vi "GetTau Delay ms.vi"(8 "error in (no error)":errorcluster, 11 "reference in":refnum<class "Force Curve_tdms.lvclass">) -> (0 "error out":errorcluster, 2 "Tau Delay ms":dbl=2.0 format="%#_13g", 3 "reference out":refnum<class "Force Curve_tdms.lvclass">)   [LabVIEW 2019, in "Force Curve_tdms.lvclass"]
uses:
  Force Curve_tdms.lvclass
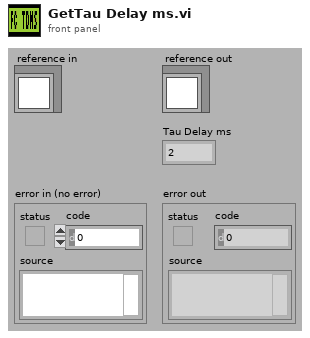
[diagram p1: front panel]
types:
  T1 = typedef "Force Curve_tdms.lvclass/ObjectAttributesRef.ctl" = refnum<data-value>
  T2 = typedef "Force Curve_tdms.lvclass/ObjectAttributes.ctl" = cluster{"MyAttribute":dbl, "Processed data":waveform(dbl)[], "Fcurve Raw Metadata":T3, "Fcurve Metadata":T4, "Fcurve index":T5, "Tau Delay (ms)":dbl, "Contact Spread of dev":dbl, "Fcurve":T6}
  T3 = typedef "TDMS_DataHandler.lvclass/Fcurve Meta data.ctl" = cluster{"property names":string[], "property values":variant[]}
  T4 = typedef "Force Curve_tdms.lvclass/Fcurve Meta data analysis.ctl" = cluster{"dt (us)":dbl, "Dec Factor":dbl, "Z piezo Sensitivity (nm/V)":dbl, "K (N/m)":dbl, "Sp (V)":dbl, "Contact (ms)":dbl, "Zpos contact":dbl, "Vel_app (nm/s)":dbl, "Vel_ret (nm/s)":dbl, "deltaV (nm)":dbl, "Def_V0 (v)":dbl, "Decimating Factor":dbl}
  T5 = typedef "Force Curve_tdms.lvclass/Fcurve Index .ctl" = cluster{"Setpoint index":i32, "Max force index":i32, "Contact point index":i32, "Appoach indices":cluster{"Start":i32, "End":i32}, "Contact indices":cluster{"Start":i32, "End":i32}, "Retract indices":cluster{"Start":i32, "End":i32}}
  T6 = typedef "Force Curve_tdms.lvclass/Force Curve data.ctl" = cluster{"Approach":cluster{"X":dbl[], "Y":dbl[]}, "Contact":cluster{"X":dbl[], "Y":dbl[]}, "Retract":cluster{"X":dbl[], "Y":dbl[]}}
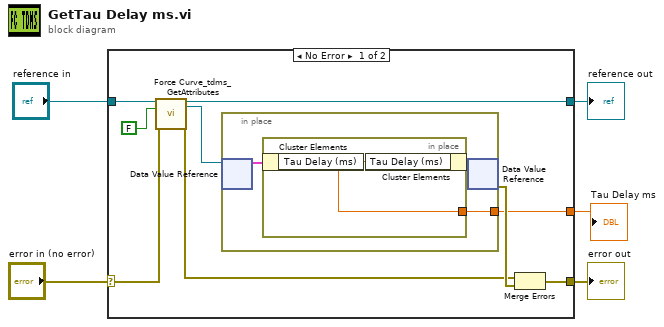
[diagram p0: block diagram]
diagram:
  n1 = case shown="No Error" "error in (no error)" {
    selector: "error in (no error)" -> [w14 w20]
    tunnel: [w8 w20] -> w4
    tunnel: [w13 w19] -> w2
    tunnel: "reference in" -> [w12 w19]
    tunnel: [w6 _] -> w1
    frame No Error {
      n2 = call "Force Curve_tdms_GetAttributes.vi"("reference in"=w12, "return data? (T)"=FALSE, "error in (no error)"=w14) -> ("reference out"=w13:refnum<class "Force Curve_tdms.lvclass">, "attributes ref"=w7:T1, "error out"=w9:errorcluster)  [unwired: 13 in, 1 out]
      n3 = in-place {
        in-place-border: [w15] -> w6
        n4 = in-place-dvr #1(w7) -> (w16:T2)  [unwired: 1 out]
        n5 = in-place {
          in-place-border: [w18] -> w15
          n6 = in-place-cluster #2(w16) -> ("Tau Delay (ms)"=w18:dbl)
          n7 = in-place-cluster #2("Tau Delay (ms)"=w18) -> (w17:T2)
        }
        n8 = in-place-dvr #1(w17) -> (w10:errorcluster)  [unwired: 1 out]
      }
      n9 = Merge Errors(w9, w10) -> (w8:errorcluster)
    }
    frame Error {
    }
  }
  "error out" <- w4
  "reference out" <- w2
  "Tau Delay ms" <- w1
